vi "falling places.vi"(9 "Size":dbl, 10 "Piece Layer":dbl[](array[numeric]), 11 "Terrain":dbl[](array[numeric])) -> (1 "Found":bool, 3 "Falling places":i32, 8 "rotate num":dbl)   [LabVIEW 2018]
panel:
  out "Boolean":bool
  out "Numeric":dbl
  out "element 2":dbl
  out "Array 2":dbl[](array[numeric])
  out "element":dbl
  out "Index 2":dbl
  out "Array":dbl[](array[numeric])
  out "Index":dbl
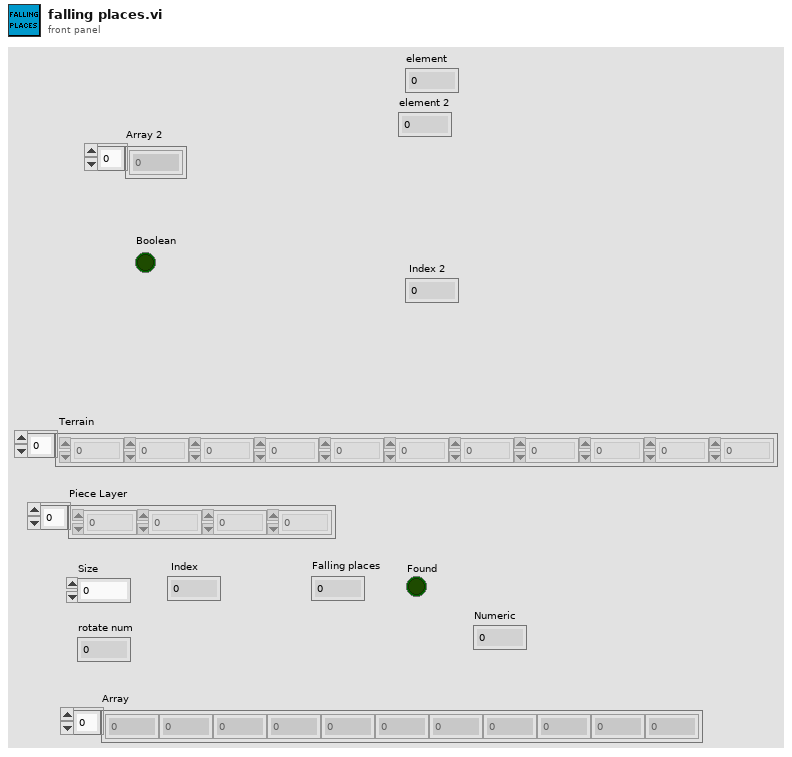
[diagram p1: front panel]
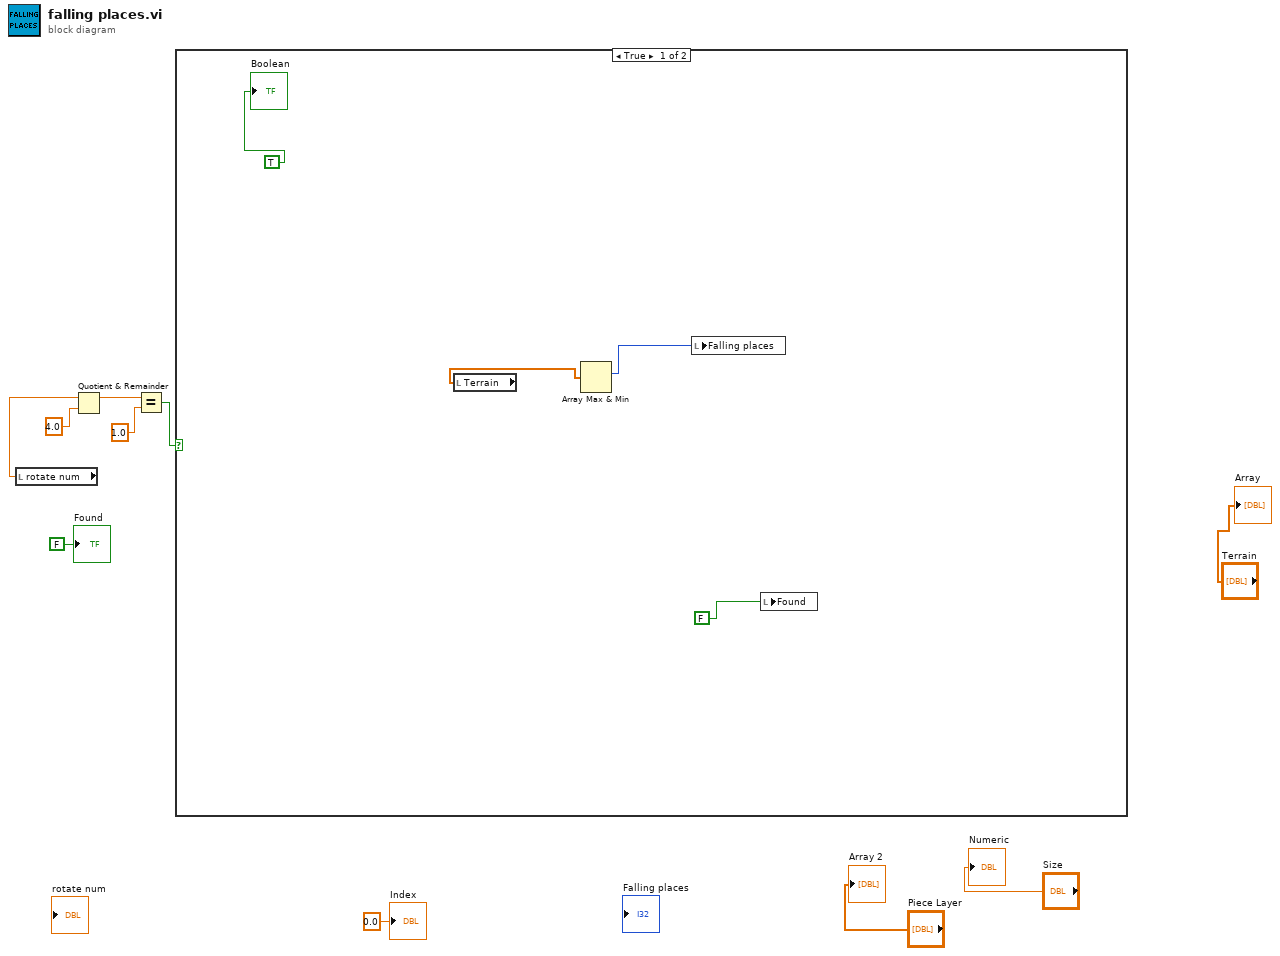
[diagram p0: block diagram]
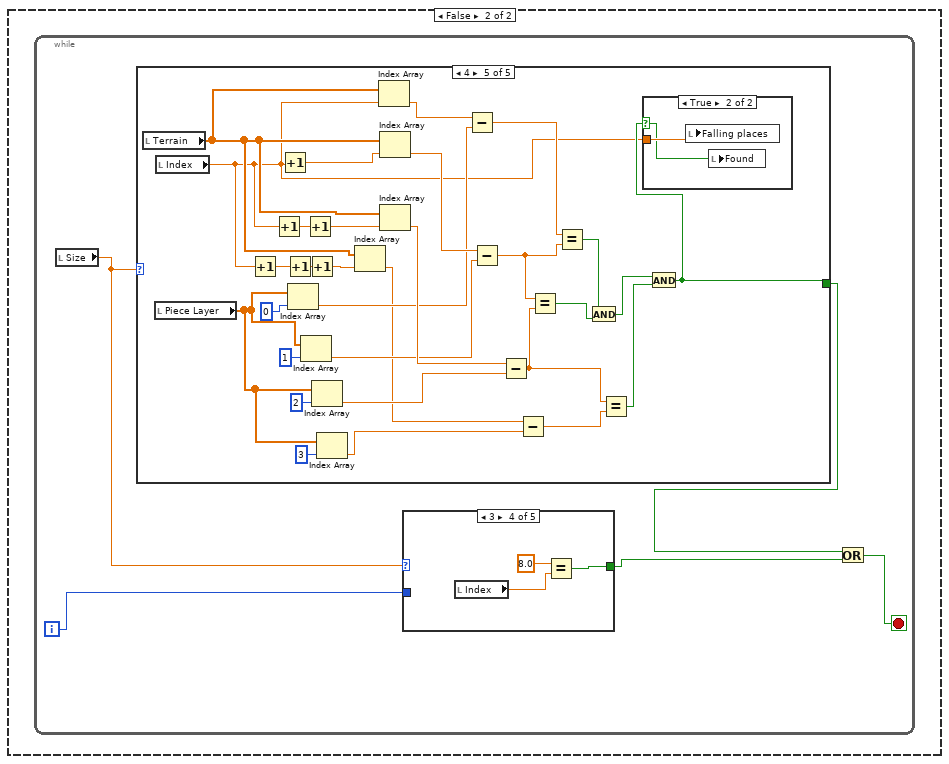
[diagram p2: hidden frame]
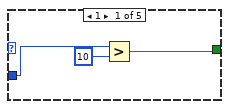
[diagram p3: hidden frame]
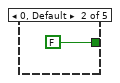
[diagram p4: hidden frame]
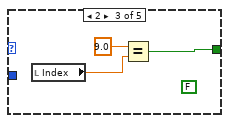
[diagram p5: hidden frame]
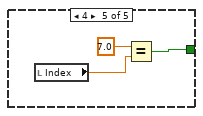
[diagram p6: hidden frame]
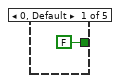
[diagram p7: hidden frame]
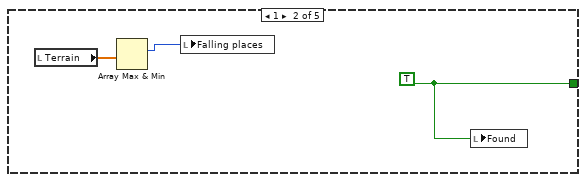
[diagram p8: hidden frame]
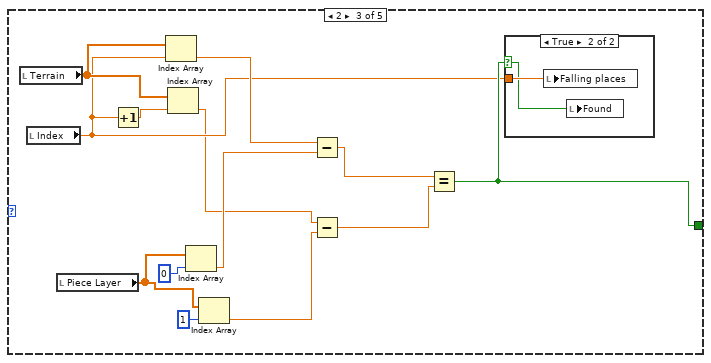
[diagram p9: hidden frame]
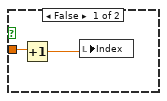
[diagram p10: hidden frame]
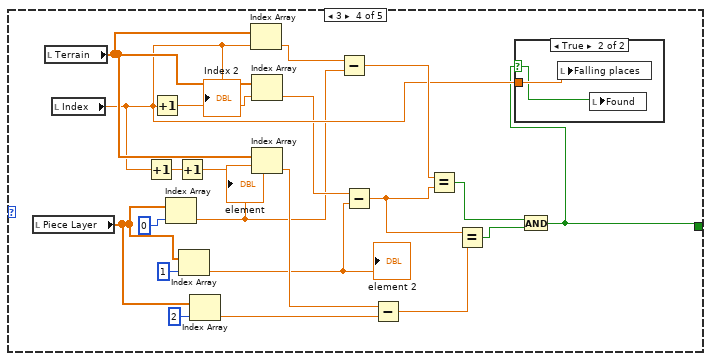
[diagram p11: hidden frame]
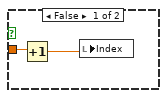
[diagram p12: hidden frame]
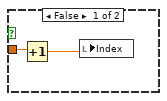
[diagram p13: hidden frame]
diagram:
  n1 = local read "rotate num"() -> (w5:dbl)
  n2 = Quotient & Remainder(x=w5, y=4.0) -> (x-y*floor(x/y)=w2:dbl)  [unwired: 1 out]
  n3 = Equal?(x=w2, y=1.0) -> (x = y?=w1:bool)
  n4 = case shown="True" w1 {
    frame True {
      n5 = local read "Terrain"() -> (w12:dbl[])
      n6 = Array Max & Min(array=w12) -> (max index (indices)=w13:i32)  [unwired: 3 out]
      n7 = local write "Falling places"(w13) -> ()
      n8 = local write "Found"(FALSE ("Found")) -> ()
      "Boolean" <- TRUE
    }
    frame False {
      n9 = while {
        i -> [w16]
        stop <- w18 stop-if-true
        n10 = local read "Size"() -> (w17:dbl)
        n11 = case shown="4" w17 {
          tunnel: [FALSE w34 w41 w59 w100] -> w19
          frame 0, Default {
          }
          frame 1 {
            w34 = TRUE
            n12 = local read "Terrain"() -> (w36:dbl[])
            n13 = Array Max & Min(array=w36) -> (max index (indices)=w35:i32)  [unwired: 3 out]
            n14 = local write "Falling places"(w35) -> ()
            n15 = local write "Found"(w34) -> ()
          }
          frame 2 {
            n16 = local read "Terrain"() -> (w49:dbl[])
            n17 = local read "Index"() -> (w40:dbl)
            n18 = local read "Piece Layer"() -> (w48:dbl[])
            n19 = Increment(x=w40) -> (x+1=w42:dbl)
            n20 = Index Array(array=w49, index=w40) -> (element=w45:dbl)
            n21 = Index Array(array=w49, index=w42) -> (element=w38:dbl)
            n22 = Index Array(array=w48, index=0) -> (element=w39:dbl)
            n23 = Index Array(array=w48, index=1) -> (element=w37:dbl)
            n24 = Subtract(x=w45, y=w39) -> (x-y=w44:dbl)
            n25 = Subtract(x=w38, y=w37) -> (x-y=w43:dbl)
            n26 = Equal?(x=w44, y=w43) -> (x = y?=w41:bool)
            n27 = case shown="True" w41 {
              selector: w41 -> [_ w52]
              tunnel: w40 -> [w51 w53]
              frame False {
                n28 = Increment(x=w51) -> (x+1=w50:dbl)
                n29 = local write "Index"(w50) -> ()
              }
              frame True {
                n30 = local write "Falling places"(w53) -> ()
                n31 = local write "Found"(w52) -> ()
              }
            }
          }
          frame 3 {
            n32 = local read "Piece Layer"() -> (w66:dbl[])
            n33 = local read "Terrain"() -> (w69:dbl[])
            n34 = local read "Index"() -> (w68:dbl)
            "Index 2" <- w68
            n35 = Increment(x=w68) -> (x+1=w55:dbl)
            n36 = Increment(x=w68) -> (x+1=w70:dbl)
            n37 = Index Array(array=w66, index=0) -> (element=w57:dbl)
            "element" <- w57
            n38 = Increment(x=w55) -> (x+1=w54:dbl)
            n39 = Index Array(array=w66, index=1) -> (element=w56:dbl)
            "element 2" <- w56
            n40 = Index Array(array=w66, index=2) -> (element=w65:dbl)
            n41 = Index Array(array=w69, index=w68) -> (element=w72:dbl)
            n42 = Index Array(array=w69, index=w70) -> (element=w58:dbl)
            n43 = Index Array(array=w69, index=w54) -> (element=w67:dbl)
            n44 = Subtract(x=w72, y=w57) -> (x-y=w71:dbl)
            n45 = Subtract(x=w58, y=w56) -> (x-y=w62:dbl)
            n46 = Subtract(x=w67, y=w65) -> (x-y=w63:dbl)
            n47 = Equal?(x=w71, y=w62) -> (x = y?=w61:bool)
            n48 = Equal?(x=w62, y=w63) -> (x = y?=w60:bool)
            n49 = And(x=w61, y=w60) -> (x .and. y?=w59:bool)
            n50 = case shown="True" w59 {
              selector: w59 -> [_ w77]
              tunnel: w68 -> [w76 w78]
              frame False {
                n51 = Increment(x=w76) -> (x+1=w75:dbl)
                n52 = local write "Index"(w75) -> ()
              }
              frame True {
                n53 = local write "Falling places"(w78) -> ()
                n54 = local write "Found"(w77) -> ()
              }
            }
          }
          frame 4 {
            n55 = local read "Terrain"() -> (w92:dbl[])
            n56 = local read "Piece Layer"() -> (w94:dbl[])
            n57 = local read "Index"() -> (w91:dbl)
            n58 = Increment(x=w91) -> (x+1=w88:dbl)
            n59 = Increment(x=w91) -> (x+1=w96:dbl)
            n60 = Increment(x=w91) -> (x+1=w104:dbl)
            n61 = Increment(x=w88) -> (x+1=w90:dbl)
            n62 = Index Array(array=w94, index=0) -> (element=w98:dbl)
            n63 = Index Array(array=w94, index=1) -> (element=w97:dbl)
            n64 = Increment(x=w96) -> (x+1=w95:dbl)
            n65 = Increment(x=w90) -> (x+1=w89:dbl)
            n66 = Index Array(array=w94, index=2) -> (element=w102:dbl)
            n67 = Index Array(array=w94, index=3) -> (element=w93:dbl)
            n68 = Index Array(array=w92, index=w89) -> (element=w87:dbl)
            n69 = Index Array(array=w92, index=w91) -> (element=w106:dbl)
            n70 = Index Array(array=w92, index=w104) -> (element=w99:dbl)
            n71 = Index Array(array=w92, index=w95) -> (element=w103:dbl)
            n72 = Subtract(x=w106, y=w98) -> (x-y=w105:dbl)
            n73 = Subtract(x=w99, y=w97) -> (x-y=w82:dbl)
            n74 = Subtract(x=w103, y=w102) -> (x-y=w83:dbl)
            n75 = Subtract(x=w87, y=w93) -> (x-y=w85:dbl)
            n76 = Equal?(x=w82, y=w83) -> (x = y?=w81:bool)
            n77 = Equal?(x=w105, y=w82) -> (x = y?=w80:bool)
            n78 = And(x=w80, y=w81) -> (x .and. y?=w79:bool)
            n79 = Equal?(x=w83, y=w85) -> (x = y?=w84:bool)
            n80 = And(x=w79, y=w84) -> (x .and. y?=w100:bool)
            n81 = case shown="True" w100 {
              selector: w100 -> [_ w111]
              tunnel: w91 -> [w110 w112]
              frame False {
                n82 = Increment(x=w110) -> (x+1=w109:dbl)
                n83 = local write "Index"(w109) -> ()
              }
              frame True {
                n84 = local write "Falling places"(w112) -> ()
                n85 = local write "Found"(w111) -> ()
              }
            }
          }
        }
        n86 = case shown="3" w17 {
          tunnel: [w20 FALSE w24 w27 w30] -> w15
          tunnel: w16 -> [w22 _ _ _ _]
          frame 1 {
            n87 = Greater?(x=w22, y=10) -> (0:w20:bool)
          }
          frame 0, Default {
          }
          frame 2 {
            (unwired) FALSE
            n88 = local read "Index"() -> (w26:dbl)
            n89 = Equal?(x=9.0, y=w26) -> (x = y?=w24:bool)
          }
          frame 3 {
            n90 = local read "Index"() -> (w29:dbl)
            n91 = Equal?(x=8.0, y=w29) -> (x = y?=w27:bool)
          }
          frame 4 {
            n92 = local read "Index"() -> (w32:dbl)
            n93 = Equal?(x=7.0, y=w32) -> (x = y?=w30:bool)
          }
        }
        n94 = Or(x=w19, y=w15) -> (x .or. y?=w18:bool)
      }
    }
  }
  "Found" <- FALSE ("Found")
  "Index" <- 0.0 ("Index")
  "Array" <- "Terrain"
  "Array 2" <- "Piece Layer"
  "Numeric" <- "Size"
